vi "FileStream Close.vi"(8 "error in (no error)":errorcluster, 11 "reference":refnum<k24>) -> (0 "error out":errorcluster)   [LabVIEW 2020, in "File Stream.lvlib"]
doc: "Closes the current stream and releases any resources."
uses:
  File Stream.lvlib
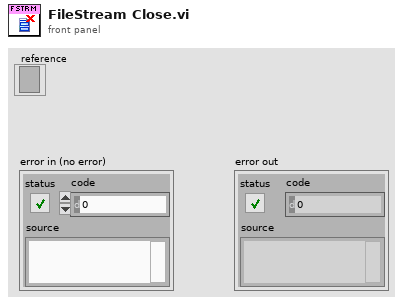
[diagram p1: front panel]
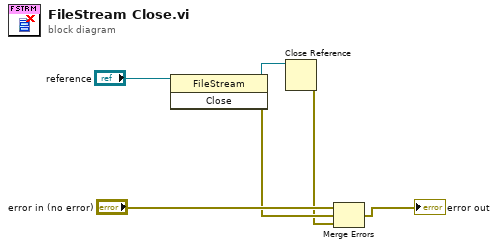
[diagram p0: block diagram]
diagram:
  n1 = invoke class="FileStream" method="Close"(reference="reference") -> (reference out=w6:refnum<k24>, error out=w2:errorcluster)  [unwired: 2 in, 1 out]
  n2 = Close Reference(reference=w6) -> (error out=w1:errorcluster)  [unwired: 1 in]
  n3 = Merge Errors("error in (no error)", w2, w1) -> (→"error out":errorcluster)
